vi "Test.vi"   [LabVIEW 2018, in "Scripts.lvlib"]
uses:
  Scripts.lvlib
  <vilib>/Field R&D Services/Labricator/Toolkit/Labricator.lvlib
  <vilib>/addons/_JKI Toolkits/Caraya/classes/Test/Test.lvclass
  tests/Tests.lvlib
panel:
  # "Overview: Runs all of tests this project\nRequirements: LabVIEW, Caraya Unit Test Framework \nInstructions: Run this VI.\n\nThis VI runs all of the integration and unit tests."
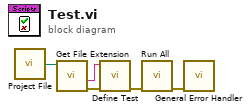
[diagram p0: block diagram]
diagram:
  n1 = call <vilib>:"Project File.vi"() -> ("Project File"=w5:path)
  n2 = call <vilib>:"Get File Extension.vi"("file"=w5) -> ("error out"=w4:errorcluster, "filename without extension"=w3:string)  [unwired: 6 in, 3 out]
  n3 = call <vilib>:"Define Test.vi"("error in (no error)"=w4, "Label (VI Title)"=w3) -> ("error out"=w2:errorcluster)  [unwired: 9 in]
  n4 = call "Run All.vi"("Error In"=w2) -> ("Error Out"=w1:errorcluster)  [unwired: 10 in]
  n5 = call <vilib>:"General Error Handler.vi"("error in (no error)"=w1) -> ()  [unwired: 10 in, 5 out]
